vi "omicron-pressure-logger-v2017-03-13.vi"() -> ()   [LabVIEW 2016]
uses:
  <vilib>/addons/h5labview2/file/H5Fmode.ctl
  <vilib>/NI/Modbus Library/API/Wrapper/Create Serial Master.vi
  <vilib>/NI/Modbus Library/API/Master/Modbus Master.lvclass
  <vilib>/NI/Modbus Library/API/Wrapper/API Main.lvlib
  <vilib>/addons/h5labview2/file/H5F.lvlib
  <vilib>/addons/h5labview2/dataset/H5D.lvlib
panel:
  in  "quit":bool
  out "Waveform Chart":dynamicdata(graph)
  out "oil pump":dbl
  out "lt":dbl format="%_3e"
  out "prep":dbl caption="PREP" format="%_3e"
  # "(mbar)"
  # "(mbar)"
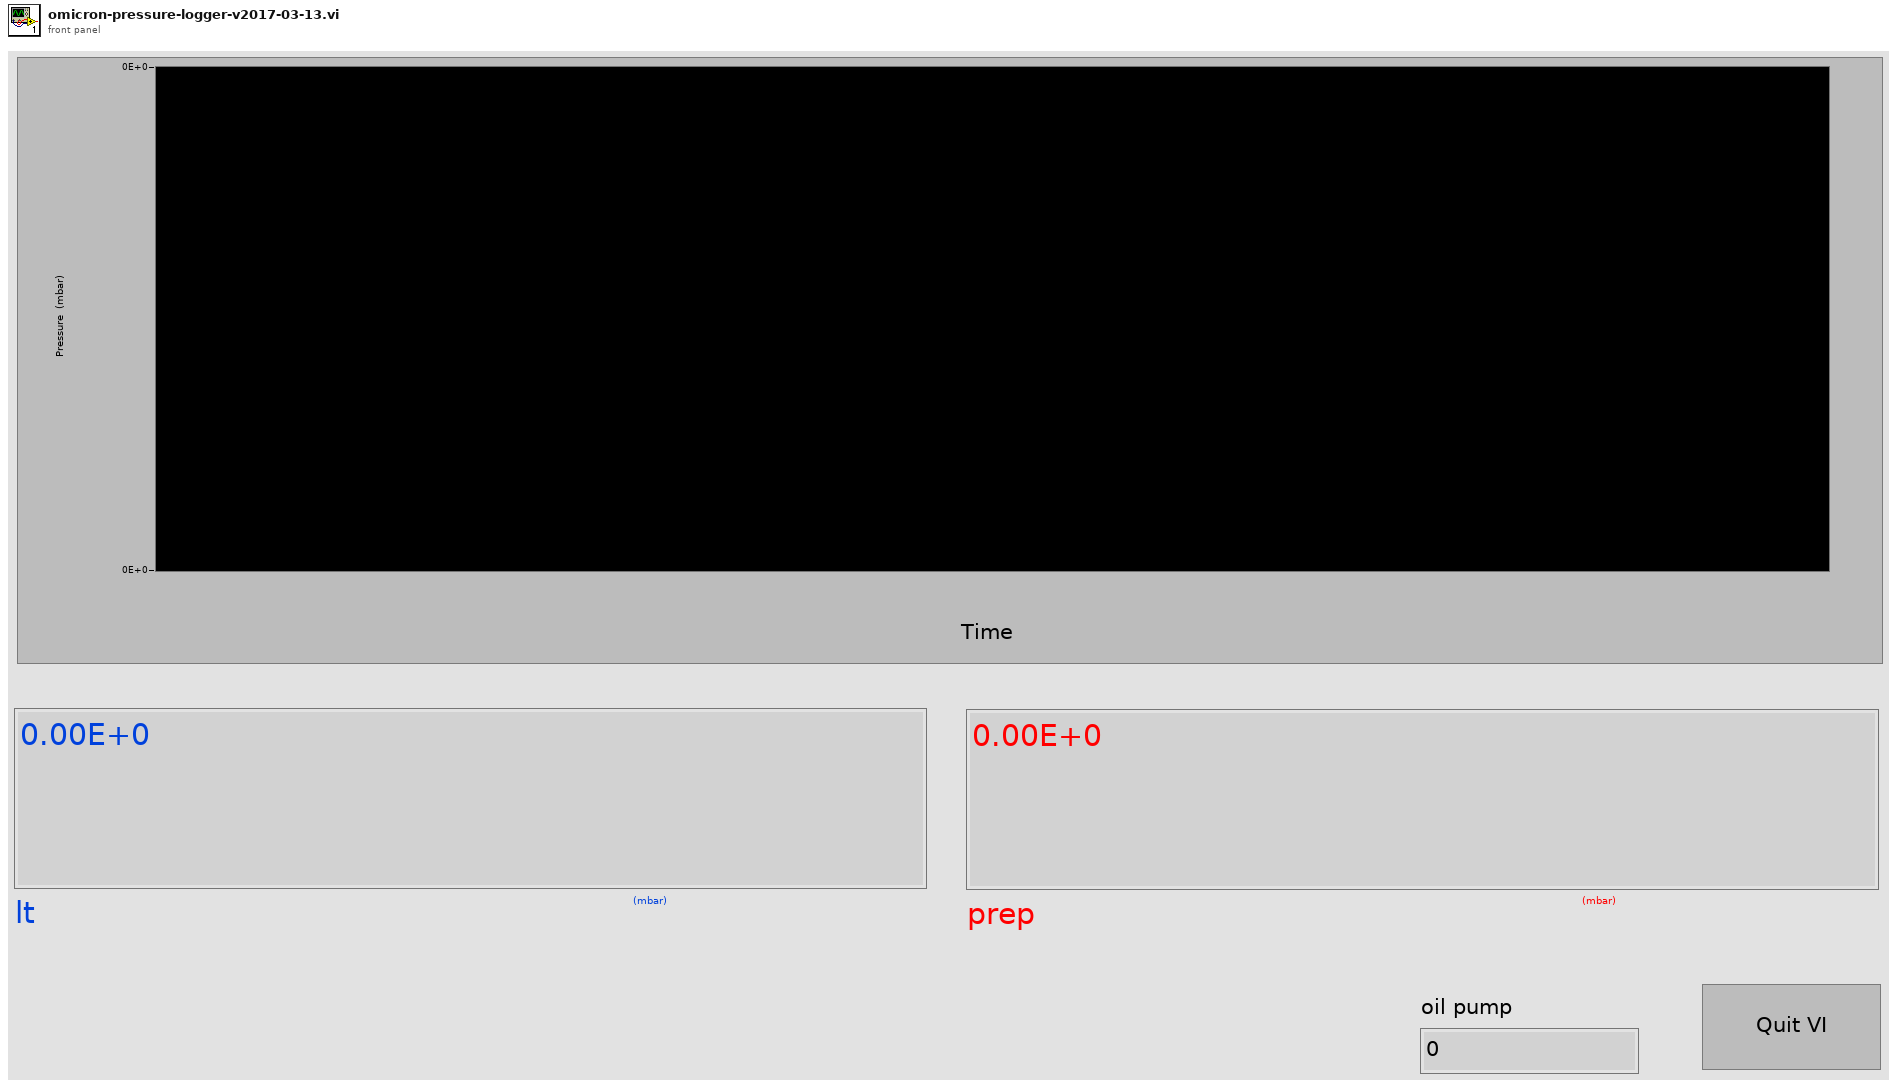
[diagram p1: front panel]
types:
  T1 = typedef "H5F.lvlib/H5Fmode.ctl" = enum16{"read-only", "read-write", "overwrite", "create new", "open or create"}
  T2 = enum16{"open", "replace", "create", "open or create", "replace or create", "replace or create with confirmation"}
  T3 = typedef "hid_t.ctl" = i32
  T4 = cluster{"timestamp":timestamp, "prep":dbl, "lt":dbl, "oil pump":dbl}
  T5 = cluster{"timestamp":timestamp, "prep":dbl, "lt":dbl, "oil pump":dbl}[]
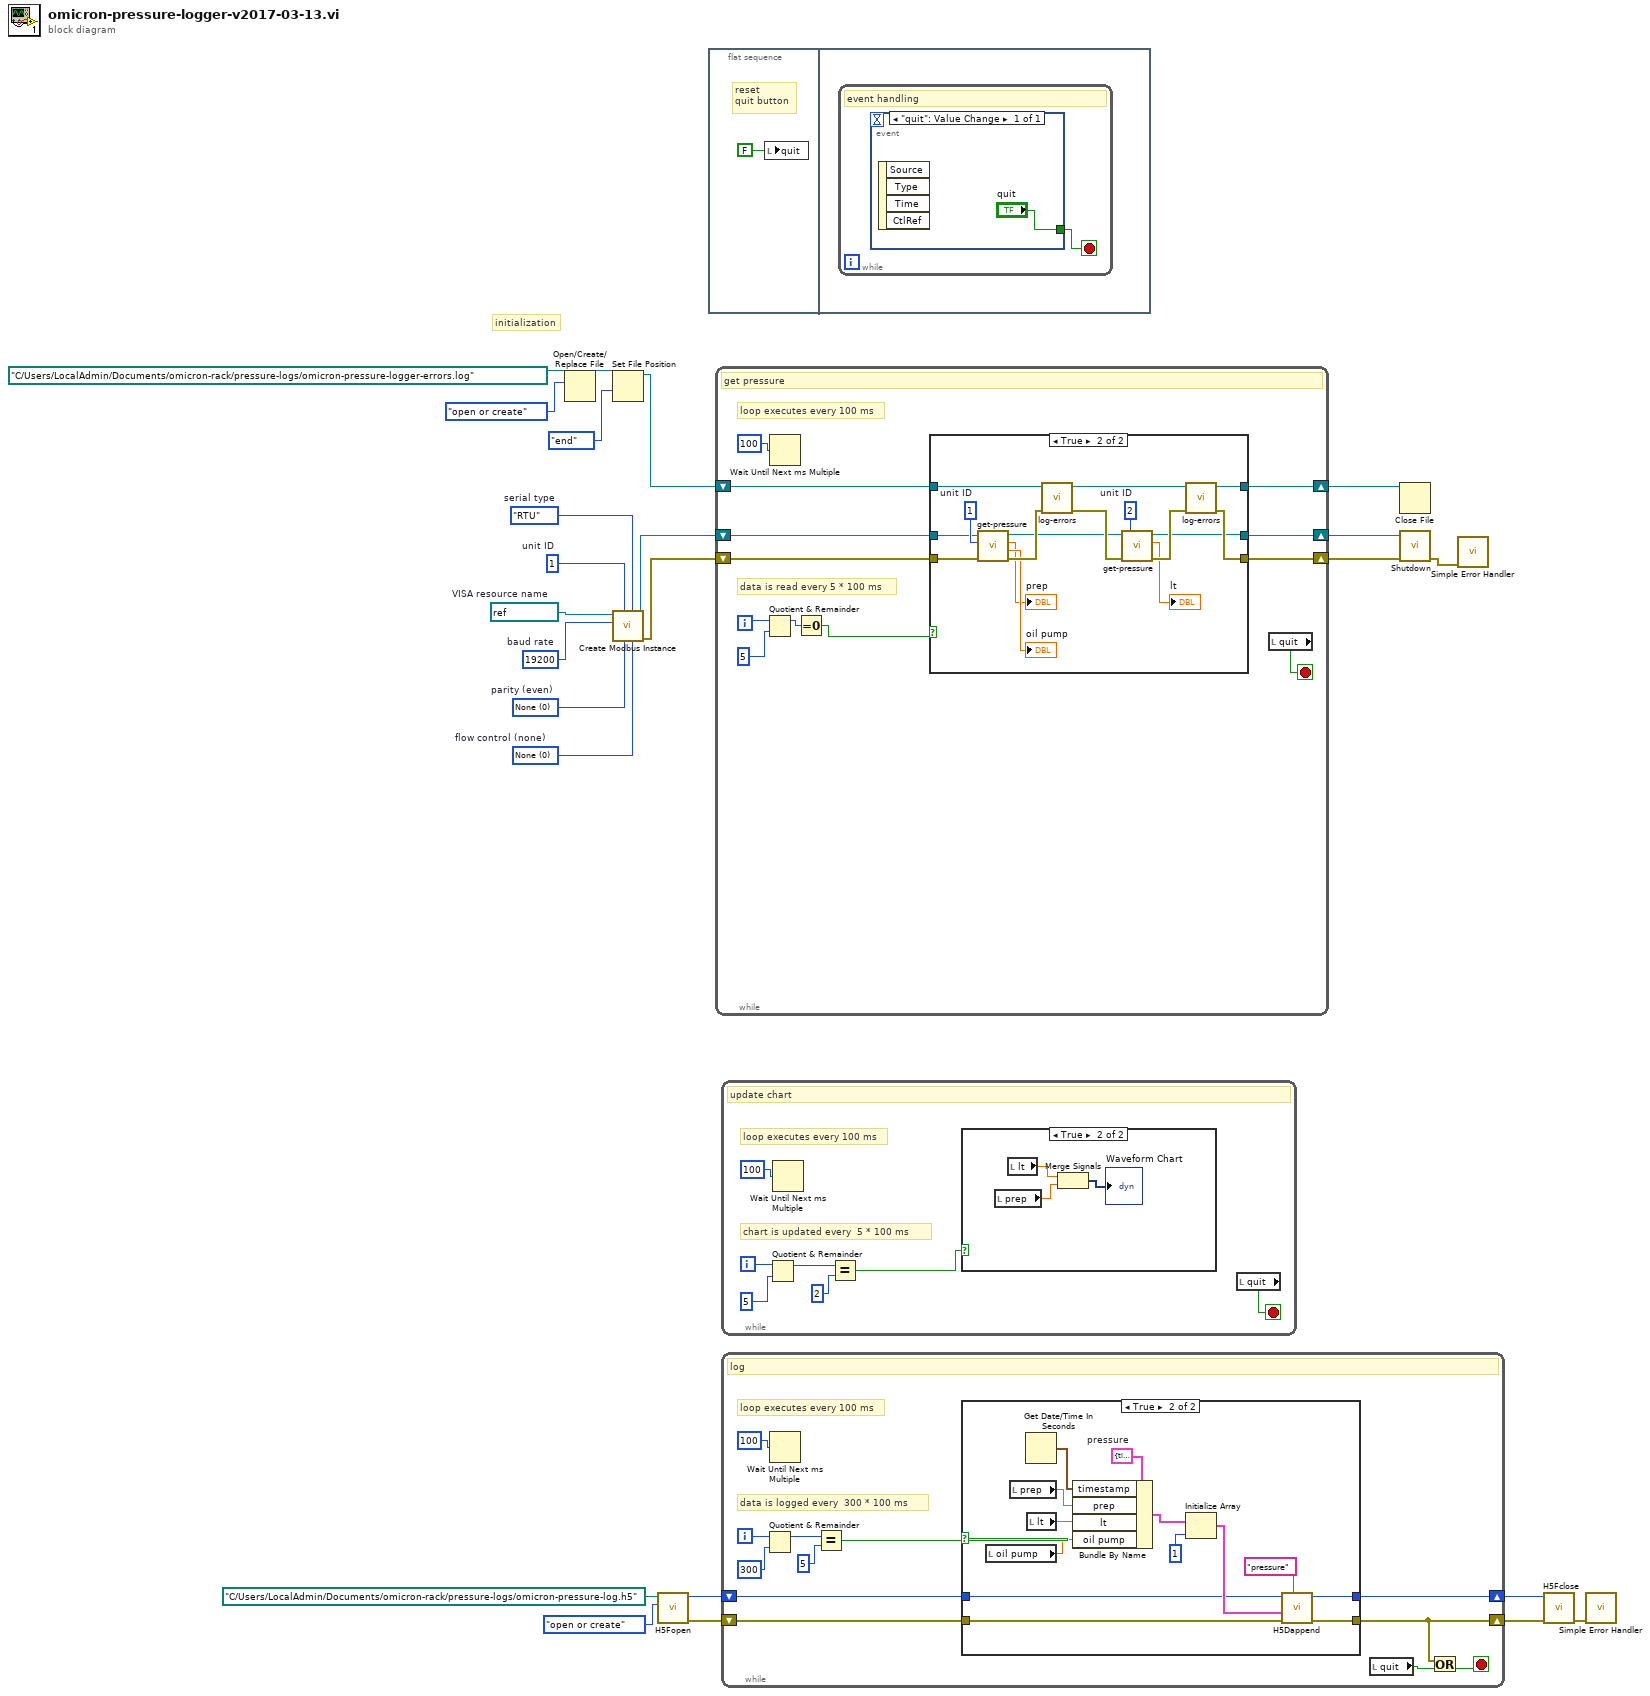
[diagram p0: block diagram]
diagram:
  w14 = u16 0 items=["None", "XON/XOFF", "RTS/CTS", "XON/XOFF & RTS/CTS", "DTR/DSR", "XON/XOFF & DTR/DSR"]  # flow control (none)
  w15 = u16 0 items=["None", "Odd", "Even", "Mark", "Space"]  # parity (even)
  w18 = u32 19200  # baud rate
  w19 = refnum<visa-resource-name> "COM11"  # VISA resource name
  w17 = u8 1  # unit ID
  w16 = enum16{"RTU", "ASCII"}."RTU"  # serial type
  # "initialization"
  n1 = Open/Create/Replace File(file path (use dialog)=path "C:/Users/LocalAdmin/Documents/omicron-rack/pressure-logs/omicron-pressure-logger-errors.log" ("Path"), operation (0:open)=T2."open or create") -> (refnum out=w11:refnum<file>)  [unwired: 4 in, 2 out]
  n2 = Set File Position(refnum=w11, from (0:start)=enum16{"start", "end", "current"}."end") -> (refnum out=w20:refnum<file>)  [unwired: 2 in, 1 out]
  n3 = call-poly <vilib>:"Create Modbus Instance.vi"("flow control (none)"=w14, "serial type"=w16, "parity (even)"=w15, "unit ID"=w17, "baud rate"=w18, "VISA resource name"=w19) -> ("error out"=w23:errorcluster, "serial master instance"=w24:refnum<class "Modbus Master.lvclass">)  [unwired: 4 in]
  n4 = call <vilib>:"H5Fopen.vi"("mode (read-only)"=H5Fmode."open or create", "path"=path "C:/Users/LocalAdmin/Documents/omicron-rack/pressure-logs/omicron-pressure-log.h5") -> ("error out"=w5:errorcluster, "ref out"=w6:T3)  [unwired: 8 in]
  n5 = flat-sequence {
    frame #0 {
      # "reset\nquit button"
      n6 = local write "quit"(FALSE) -> ()
    }
    frame #1 {
      n7 = while {
        stop <- w26 stop-if-true
        # "event handling"
        n8 = event shown="[0] \"quit\": Value Change" {
          selector: _ -> [_]
          dyn-events: _ -> [_]
          timeout: _ -> [_]
          tunnel: ["quit"] -> w26
          event "quit": Value Change {
            n9 = event-data() -> ()  [unwired: 1 in, 4 out]
          }
        }
      }
    }
  }
  n10 = while {
    shift-right: [w29] -> w22
    shift-left: w24 -> [w32]
    shift-right: [w28] -> w21
    shift-left: w23 -> [w31]
    shift-right: [w30] -> w9
    shift-left: w20 -> [w33]
    i -> [w34]
    stop <- w39 stop-if-true
    # "data is read every 5 * 100 ms"
    # "loop executes every 100 ms"
    # "get pressure"
    n11 = Quotient & Remainder(x=w34, y=5) -> (x-y*floor(x/y)=w36:i32)  [unwired: 1 out]
    n12 = Wait Until Next ms Multiple(millisecond multiple=u32 100 ("milliseconds to wait")) -> ()  [unwired: 1 out]
    n13 = Equal To 0?(x=w36) -> (x = 0?=w35:bool)
    n14 = case shown="True" w35 {
      tunnel: w33 -> [w42 w48]
      tunnel: w32 -> [w40 w47]
      tunnel: w31 -> [w41 w46]
      tunnel: [w42 w45] -> w30
      tunnel: [w41 w44] -> w28
      tunnel: [w40 w43] -> w29
      frame False {
      }
      frame True {
        w51 = u8 2  # unit ID
        w50 = u8 1  # unit ID
        n15 = call "get-pressure.vi"("error in"=w46, "unit ID"=w50, "Modbus instance in"=w47) -> ("error out"=w55:errorcluster, "Pirani"=→"oil pump":sgl, "Ion Gauge Pressure"=→"prep":sgl, "Modbus instance out"=w49:refnum<class "Modbus Master.lvclass">)  [unwired: 5 in]
        n16 = call "log-errors.vi"("error in (no error)"=w55, "refnum in"=w48) -> ("error out"=w56:errorcluster, "refnum"=w58:refnum<file>)  [unwired: 8 in]
        n17 = call "get-pressure.vi"("error in"=w56, "unit ID"=w51, "Modbus instance in"=w49) -> ("error out"=w57:errorcluster, "Ion Gauge Pressure"=→"lt":sgl, "Modbus instance out"=w43:refnum<class "Modbus Master.lvclass">)  [unwired: 5 in, 1 out]
        n18 = call "log-errors.vi"("error in (no error)"=w57, "refnum in"=w58) -> ("error out"=w44:errorcluster, "refnum"=w45:refnum<file>)  [unwired: 8 in]
      }
    }
    n19 = local read "quit"() -> (w39:bool)
  }
  n20 = while {
    i -> [w62]
    stop <- w65 stop-if-true
    # "chart is updated every  5 * 100 ms"
    # "loop executes every 100 ms"
    # "update chart"
    n21 = Quotient & Remainder(x=w62, y=5) -> (x-y*floor(x/y)=w60:i32)  [unwired: 1 out]
    n22 = Wait Until Next ms Multiple(millisecond multiple=u32 100 ("milliseconds to wait")) -> ()  [unwired: 1 out]
    n23 = Equal?(x=w60, y=2) -> (x = y?=w59:bool)
    n24 = case shown="True" w59 {
      frame False {
      }
      frame True {
        n25 = local read "prep"() -> (w66:dbl)
        n26 = local read "lt"() -> (w67:dbl)
        n27 = Merge Signals(w67, w66) -> (→"Waveform Chart":dynamicdata)
      }
    }
    n28 = local read "quit"() -> (w65:bool)
  }
  n29 = while {
    shift-right: [w73] -> w3
    shift-left: w6 -> [w75]
    shift-right: [w71] -> w2
    shift-left: w5 -> [w74]
    i -> [w77]
    stop <- w72 stop-if-true
    # "data is logged every  300 * 100 ms"
    # "loop executes every 100 ms"
    # "log"
    n30 = Quotient & Remainder(x=w77, y=300) -> (x-y*floor(x/y)=w70:i32)  [unwired: 1 out]
    n31 = Wait Until Next ms Multiple(millisecond multiple=u32 100 ("milliseconds to wait")) -> ()  [unwired: 1 out]
    n32 = Equal?(x=w70, y=5) -> (x = y?=w76:bool)
    n33 = case shown="True" w76 {
      tunnel: w75 -> [w82 w86]
      tunnel: w74 -> [w81 w85]
      tunnel: [w82 w84] -> w73
      tunnel: [w81 w83] -> w71
      frame False {
      }
      frame True {
        w94 = T4 {"timestamp"=timestamp(0 s since 1904-01-01), "prep"=0.0, "lt"=0.0, "oil pump"=0.0}  # pressure
        n34 = local read "oil pump"() -> (w91:dbl)
        n35 = local read "prep"() -> (w93:dbl)
        n36 = Get Date/Time In Seconds() -> (seconds since 1Jan1904=w95:timestamp)
        n37 = local read "lt"() -> (w92:dbl)
        n38 = Bundle By Name(cluster=w94, "timestamp"=w95, "prep"=w93, "lt"=w92, "oil pump"=w91) -> (w89:T4)
        n39 = Initialize Array(w89, 1 ("dimension size")) -> (w87:T5)
        n40 = call <vilib>:"H5Dappend.vi"("dataset name"="pressure" ("name"), "error in (no error)"=w85, "data"=w87, "ref in"=w86) -> ("error out"=w83:errorcluster, "ref out"=w84:T3)  [unwired: 4 in, 2 out]
      }
    }
    n41 = local read "quit"() -> (w80:bool)
    n42 = Or(x=w71, y=w80) -> (x .or. y?=w72:bool)
  }
  n43 = Close File(refnum=w9) -> ()  [unwired: 1 in, 2 out]
  n44 = call-dynamic "Shutdown.vi"("error in"=w21, "Modbus master in"=w22) -> ("error out"=w1:errorcluster)  [unwired: 9 in]
  n45 = call <vilib>:"Simple Error Handler.vi"("error in (no error)"=w1) -> ()  [unwired: 4 in, 5 out]
  n46 = call <vilib>:"H5Fclose.vi"("error in (no error)"=w2, "ref"=w3) -> ("error out"=w4:errorcluster)  [unwired: 9 in]
  n47 = call <vilib>:"Simple Error Handler.vi"("error in (no error)"=w4) -> ()  [unwired: 4 in, 5 out]
